vi "import_suv_vis.vi"() -> ()   [LabVIEW 2017]
panel:
  in  "stop":bool
  out "Temp F":dbl(knob) scale=0.0..100.0
  in  "Temp c":dbl(slide) scale=0.0..10.0
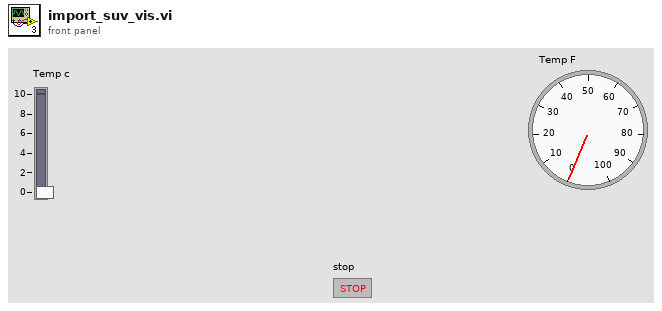
[diagram p1: front panel]
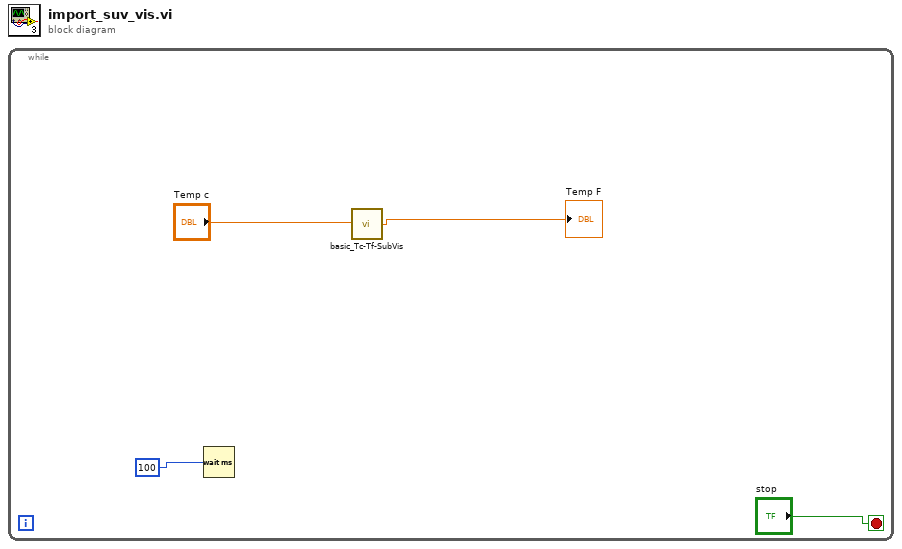
[diagram p0: block diagram]
diagram:
  n1 = while {
    stop <- "stop" stop-if-true
    n2 = Wait (ms)(milliseconds to wait=u32 100 ("millisecond timer value")) -> ()  [unwired: 1 out]
    n3 = call "basic_Tc-Tf-SubVis.vi"("Tc"="Temp c") -> ("Tf"=→"Temp F":dbl)
  }
